vi "RSZVB Trace Data To Memory.vi"(8 "error in (no error)":errorcluster {"code" format="%.0x"}, 10 "Channel (Trace) (1)":i32=1, 11 "VISA session":refnum<visa-resource-name>) -> (0 "error out":errorcluster {"code" format="%.0x"}, 3 "dup VISA session":refnum<visa-resource-name>)   [LabVIEW 2011]
doc: "This VI copies the current state of the active data trace to a memory trace. If a mathematical trace is active, the data trace associated with the mathematical trace is copied. The memory trace is named Mem<n>[<Data_Trace>] where <n> counts all data and memory traces in the active setup in chronological order, and <Data_Trace> is the name of the associated (copied) data trace. \n\nThe exact VI of the command depends on the number of memory traces associated to the active data trace:\n\n- If no memory trace is associated to the active trace, a new memory trace is generated.\n\n- If several memory traces are associated to the active trace, the current measurement data overwrites the last generated or changed memory trace. \n\nNote(s):\n\nTo copy a trace to the memory without overwriting an existing memory trace or define a memory trace name, use TRACe:COPY <memory_trc>,<data_trc>. To copy an active mathematical trace use TRACe:COPY:MATH <memory_trc>,<data_trc>.\n\nRemote-control command(s):\nCALCulate<Ch/Tr>:MATH:MEMorize"
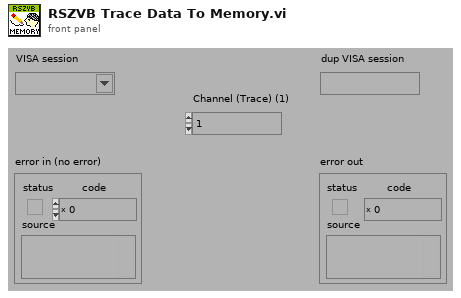
[diagram p1: front panel]
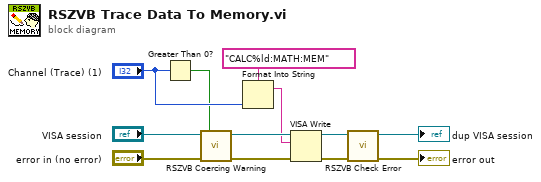
[diagram p0: block diagram]
diagram:
  n1 = Greater Than 0?(x="Channel (Trace) (1)") -> (x > 0?=w1:bool)
  n2 = call "RSZVB Coercing Warning.vi"("In Range?"=w1, "error in (no error)"="error in (no error)", "VISA session"="VISA session") -> ("error out"=w10:errorcluster, "dup VISA session"=w11:refnum<visa-resource-name>)  [unwired: 7 in]
  n3 = Format Into String(format string="CALC%ld:MATH:MEM", "Channel (Trace) (1)") -> (resulting string=w7:string)  [unwired: 2 in, 1 out]
  n4 = VISA Write(VISA resource name=w11, write buffer=w7, error in (no error)=w10) -> (VISA resource name out=w8:refnum<visa-resource-name>, error out=w9:errorcluster)  [unwired: 1 out]
  n5 = call "RSZVB Check Error.vi"("error in (no error)"=w9, "VISA session"=w8) -> ("error out"=→"error out":errorcluster, "dup VISA session"=→"dup VISA session":refnum<visa-resource-name>)  [unwired: 8 in]
